vi "Com_SECS Equipment _Format Code.vi"(1 "Formay Code":bool[](array[boolean])) -> (0 "Format Code":T1)   [LabVIEW 2016]
uses:
  Data Def/Com_SECS Equipment _Format Code.ctl
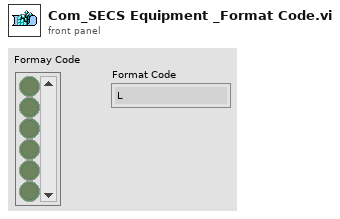
[diagram p1: front panel]
types:
  T1 = typedef "Com_SECS Equipment _Format Code.ctl" = enum16{"L", "A", "B", "Boolean", "J", "I1", "I2", "I4", "I8", "U1", "U2", "U4", "U8", "F4", "F8", "Char"}
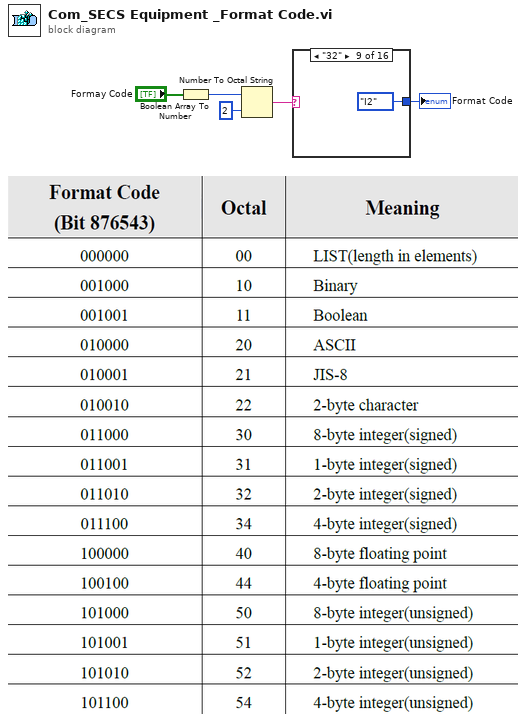
[diagram p0: block diagram]
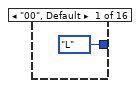
[diagram p2: hidden frame]
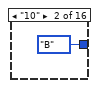
[diagram p3: hidden frame]
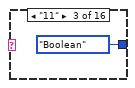
[diagram p4: hidden frame]
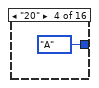
[diagram p5: hidden frame]
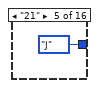
[diagram p6: hidden frame]
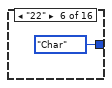
[diagram p7: hidden frame]
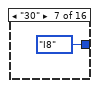
[diagram p8: hidden frame]
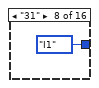
[diagram p9: hidden frame]
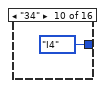
[diagram p10: hidden frame]
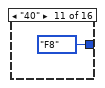
[diagram p11: hidden frame]
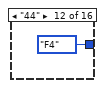
[diagram p12: hidden frame]
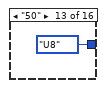
[diagram p13: hidden frame]
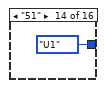
[diagram p14: hidden frame]
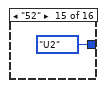
[diagram p15: hidden frame]
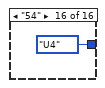
[diagram p16: hidden frame]
diagram:
  n1 = Boolean Array To Number(Boolean array="Formay Code") -> (number=w4:u32)
  n2 = Number To Octal String(1:i16 2 ("width (-)"), 2:w4) -> (0:w2:string)
  n3 = case shown="\"32\"" w2 {
    tunnel: [Com_SECS_Equipment__Format_Code."L" ("Format Code") Com_SECS_Equipment__Format_Code."B" ("Format Code") Com_SECS_Equipment__Format_Code."Boolean" ("Format Code") Com_SECS_Equipment__Format_Code."A" ("Format Code") Com_SECS_Equipment__Format_Code."J" ("Format Code") Com_SECS_Equipment__Format_Code."Char" ("Format Code") Com_SECS_Equipment__Format_Code."I8" ("Format Code") Com_SECS_Equipment__Format_Code."I1" ("Format Code") Com_SECS_Equipment__Format_Code."I2" ("Format Code") Com_SECS_Equipment__Format_Code."I4" ("Format Code") Com_SECS_Equipment__Format_Code."F8" ("Format Code") Com_SECS_Equipment__Format_Code."F4" ("Format Code") Com_SECS_Equipment__Format_Code."U8" ("Format Code") Com_SECS_Equipment__Format_Code."U1" ("Format Code") Com_SECS_Equipment__Format_Code."U2" ("Format Code") Com_SECS_Equipment__Format_Code."U4" ("Format Code")] -> w1
    frame "00", Default {
    }
    frame "10" {
    }
    frame "11" {
    }
    frame "20" {
    }
    frame "21" {
    }
    frame "22" {
    }
    frame "30" {
    }
    frame "31" {
    }
    frame "32" {
    }
    frame "34" {
    }
    frame "40" {
    }
    frame "44" {
    }
    frame "50" {
    }
    frame "51" {
    }
    frame "52" {
    }
    frame "54" {
    }
  }
  "Format Code" <- w1
